vi "Set_Parameter_Instrument (Json).vi"(8 "error in (no error)":errorcluster caption="entrée d'erreur (pas d'erreur)", 10 "Parameter (Json)":string, 11 "Show_Information en entrée":refnum<class "Wait_CloseShielding.lvclass">) -> (0 "error out":errorcluster caption="sortie d'erreur", 3 "Show_Information en sortie":refnum<class "Wait_CloseShielding.lvclass">)   [LabVIEW 2020, in "Library Test.lvlib" / "Wait_CloseShielding.lvclass"]
uses:
  Wait_CloseShielding.lvclass
  C:/Users/ngarcin/OneDrive - Altyor/Standard TB/Class/Test/Test (Default)/Test (Default).lvclass
  Wait_CloseShielding.lvclass/Wait_CloseShielding.ctl
  JSON API/JSON Value/Set from JSON string.vi
  Test/Test_Without_Instr/Test_Without_Inst.lvclass
  Instrument/Instrument (Default)/Class Instrument (Default).lvclass
  JSON API/JSON Value/JSON Value.lvclass
  JSON API/Variant JSON/Variant JSON.lvlib
  JSON API/Get Polymorphic/JSON GetSet.lvlib
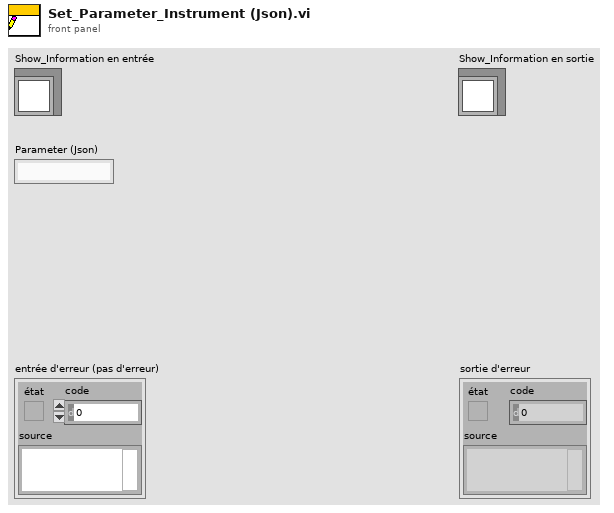
[diagram p1: front panel]
types:
  T1 = cluster{"Information_Operator":string, "Path_Picture":path, "Timeout (ms)":u64, "Function to Write":enum16{"Close", "Open"}}
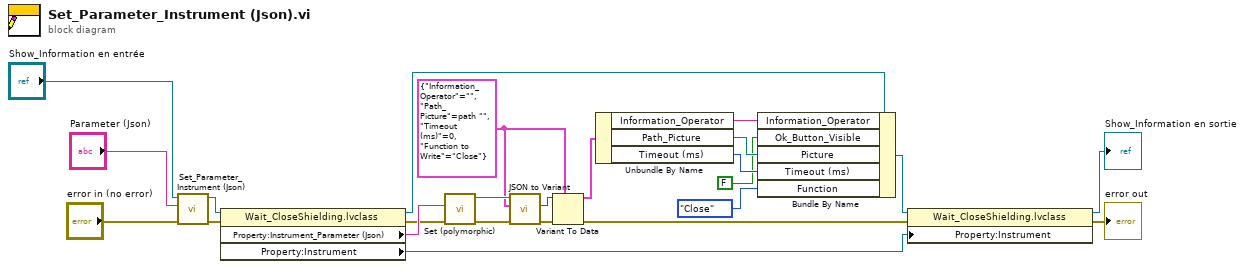
[diagram p0: block diagram]
diagram:
  w8 = T1 {"Information_Operator"="", "Path_Picture"=path "", "Timeout (ms)"=0, "Function to Write"=enum."Close"} ("Cluster des données privées de classe")
  n1 = call-parent "Set_Parameter_Instrument (Json).vi"("error in (no error)"="error in (no error)", "Parameter (Json)"="Parameter (Json)", "Test (Default) en entrée"="Show_Information en entrée") -> ("error out"=w14:errorcluster, "Test (Default) en sortie"=w15:refnum<class "Wait_CloseShielding.lvclass">)  [unwired: 7 in]
  n2 = property class="Wait_CloseShielding.lvclass"(reference=w15, error in=w14) -> (reference out=w13:refnum<class "Wait_CloseShielding.lvclass">, error out=w20:errorcluster, "Property:Instrument_Parameter (Json)"=w21:string, "Property:Instrument"=w2:refnum<class "Class Instrument (Default).lvclass">)
  n3 = call-poly "Set (polymorphic).vi"("error in (no error)"=w20, "JSON stream"=w21) -> ("error out"=w17:errorcluster, "JSON Value out"=w19:refnum<class "JSON Value.lvclass">)  [unwired: 7 in, 1 out]
  n4 = call "JSON to Variant.vi"("error in (no error)"=w17, "Variant (Data Type)"=w8, "JSON Value"=w19) -> ("error out"=w18:errorcluster, "Variant out"=w16:variant)  [unwired: 7 in]
  n5 = Variant To Data(error in=w18, type=w8, Variant=w16) -> (data=w12:T1, error out=w3:errorcluster)
  n6 = Unbundle By Name(w12) -> ("Information_Operator"=w11:string, "Path_Picture"=w10:path, "Timeout (ms)"=w9:u64)
  n7 = Bundle By Name(cluster=w13, "Information_Operator"=w11, "Ok_Button_Visible"=FALSE, "Picture"=w10, "Timeout (ms)"=w9, "Function"=enum16{"Close", "Open"}."Close") -> (w7:refnum<class "Wait_CloseShielding.lvclass">)
  n8 = property class="Wait_CloseShielding.lvclass"(reference=w7, error in=w3, "Property:Instrument"=w2) -> (reference out=→"Show_Information en sortie":refnum<class "Wait_CloseShielding.lvclass">, error out=→"error out":errorcluster)
